vi "StudentScope - Two Ch Update.vi"(9 "Samples/Graph":dbl, 10 "scope graph ref 2":refnum<vi>, 11 "scope graph ref":refnum<vi>) -> ()   [LabVIEW 2015]
doc: "This subVI updates the scope graph. It handles scaling, vertical position, and whether a channel is on or off."
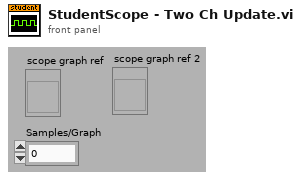
[diagram p1: front panel]
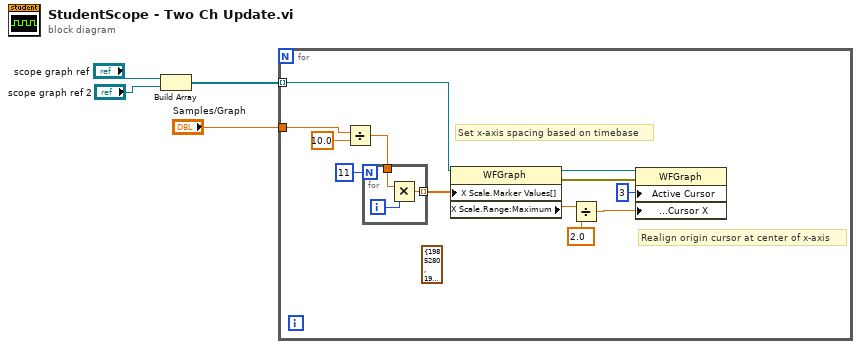
[diagram p0: block diagram]
diagram:
  n1 = Build Array("scope graph ref", "scope graph ref 2") -> (w1:refnum<vi>[])
  n2 = for {
    tunnel: "Samples/Graph" -> [w14]
    tunnel: w1 -> [w5] mode=indexing
    (unwired) cluster{u32, u32} {1985280, 1985280} ("Grid Colors")
    # "Realign origin cursor at center of x-axis"
    # "Set x-axis spacing based on timebase"
    n3 = Divide(x=w14, y=10.0) -> (x/y=w12:dbl)
    n4 = for {
      N: 11 -> [_]
      tunnel: [w18] -> w15 mode=indexing
      tunnel: w12 -> [w17]
      i -> [w19]
      n5 = Multiply(x=w17, y=w19) -> (x*y=w18:dbl)
    }
    n6 = property class="WFGraph"(reference=w5, "X Scale.Marker Values[]"=w15) -> (reference out=w9:refnum<vi>, error out=w11:errorcluster, "X Scale.Range:Maximum"=w6:dbl)  [unwired: 1 in]
    n7 = Divide(x=w6, y=2.0) -> (x/y=w7:dbl)
    n8 = property class="WFGraph"(reference=w9, error in=w11, "Active Cursor"=u32 3 ("Active Plot"), "Cursor.Cursor Position:Cursor X"=w7) -> ()  [unwired: 2 out]
  }
